vi "Steering Math.vi"() -> ()   [LabVIEW 2020]
uses:
  <vilib>/Analysis/coordinate.llb/Angle Range (Degree).ctl
  <vilib>/Analysis/coordinate.llb/Angle Units.ctl
  <vilib>/Analysis/coordinate.llb/Bisect Angle (array).vi
  <vilib>/Analysis/coordinate.llb/Angle Rotation (array).vi
  <vilib>/Analysis/coordinate.llb/Absolute Angle Difference (array).vi
  <vilib>/Analysis/coordinate.llb/Angle Rotation (scalar).vi
  <vilib>/Analysis/coordinate.llb/Wrap Angle (array).vi
  <vilib>/Analysis/coordinate.llb/Set Angle Unit.vi
  <vilib>/Analysis/coordinate.llb/Wrap Angle (scalar).vi
  <vilib>/Analysis/NI_AAL_Angle.lvlib
  <vilib>/Rock Robotics/WPI/ThirdParty/REV Robotics/REVLib/Typedef/Spark MAX Control Type.ctl
  <vilib>/Rock Robotics/WPI/ThirdParty/REV Robotics/REVLib/Typedef/Spark MAX Sensor Type.ctl
  <vilib>/Rock Robotics/WPI/ThirdParty/Phoenix-LabVIEW/Pigeon IMU/CTRE_PigeonIMU_GetYPR.vi
panel:
  out "BL Drive":dbl
  out "BR Drive":dbl
  out "FR Drive":dbl
  in  "milliseconds to wait":u32=20
  out "FL Drive":dbl
  in  "Right X":dbl
  out "Turn Left":dbl[](array[numeric])
  out "Turn Right":dbl[](array[numeric])
  out "Drive dband":dbl
  out "Steer dband":dbl
  in  "PID 550":T1={"P Gain"=0.003, "I Gain"=0.0, "D Gain"=0.006, "F Gain"=0.0, "I Zone"=0.009999999999999997, "Min Output"=-1.0, "Max Output"=1.0} {"Max Output" min=-1.0 max=1.0 step=0.01; "Min Output" min=-1.0 max=1.0 step=0.01; "I Zone" step=0.01; "F Gain" step=0.01; "D Gain" step=0.01; "I Gain" step=0.01; "P Gain" min=0.0 step=0.01}
  out "PID FL":T2(graph)
  out "FL Steer":dbl
  out "PID FR":T2(graph)
  out "FR Steer":dbl
  out "PID BL":T2(graph)
  out "BL Steer":dbl
  out "PID BR":T2(graph)
  out "BR Steer":dbl
  in  "Gyro":bool
  in  "Manual Gyro":dbl
  in  "Left X":dbl
  in  "Left Y":dbl
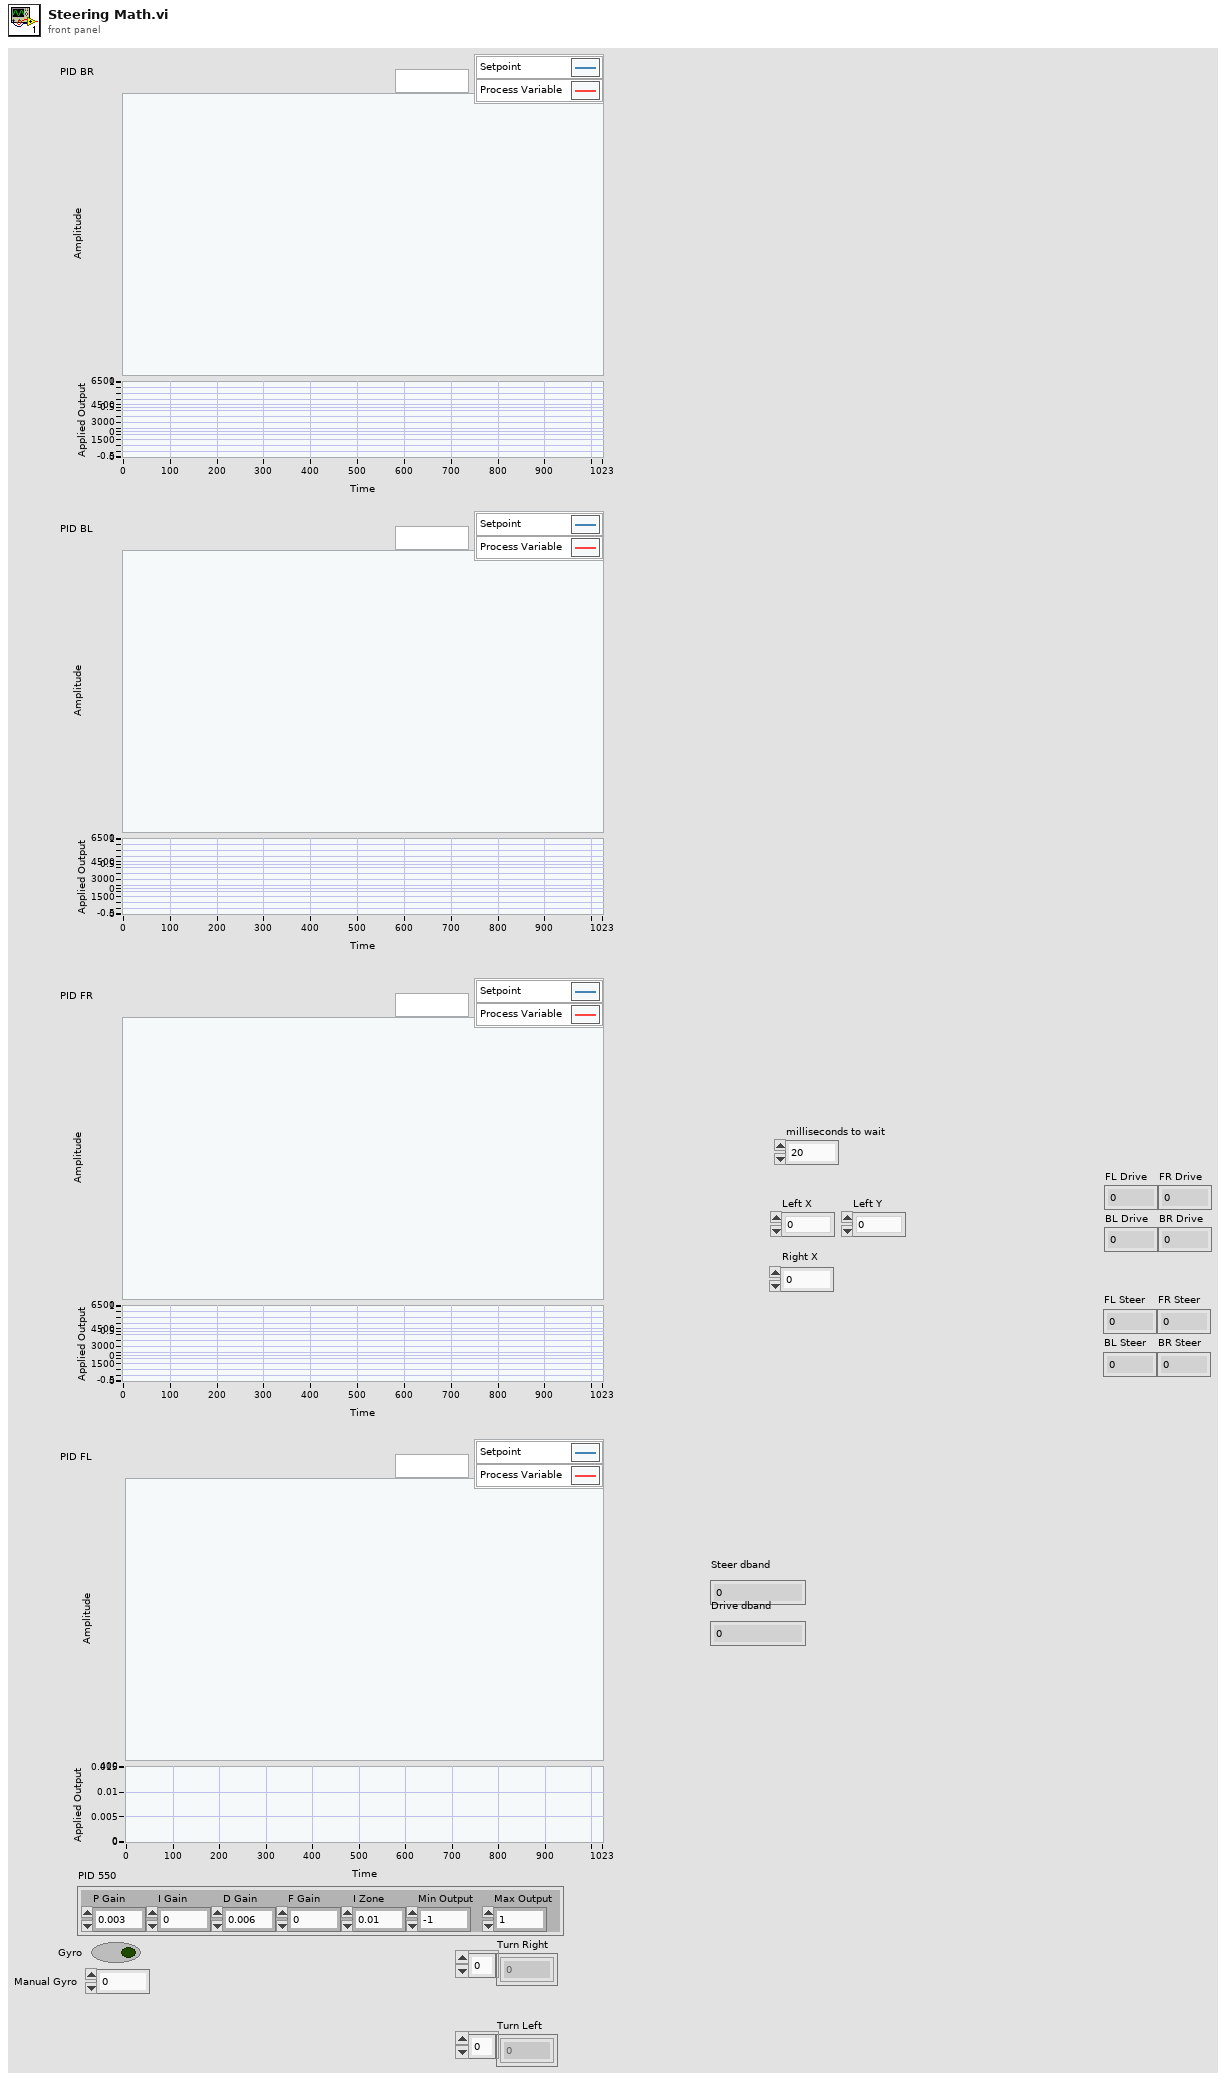
[diagram p1: front panel]
types:
  T1 = cluster{"P Gain":dbl, "I Gain":dbl, "D Gain":dbl, "F Gain":dbl, "I Zone":dbl, "Min Output":dbl, "Max Output":dbl}
  T2 = cluster{"Sensor Velocity":dbl, "Setpoint":dbl, "Applied Output":dbl}
  T3 = typedef "Spark MAX Sensor Type.ctl" = enum16{"No Sensor", "Hall Sensor", "Encoder", "-Not Available-", "Analog", "Alternate Encoder", "Duty Cycle"}
  T4 = typedef "Spark MAX Control Type.ctl" = enum16{"Percent VBus", "Voltage", "Velocity", "Position", "Smart Motion", "Current", "Smart Velocity"}
  T5 = typedef "WPI_MotorControlDeviceRef.ctl" = cluster{"DeviceStatus":errorcluster, "Type":T6, "PWM":cluster{"PWM Channel":T7, "DeadBand":T8}, "CAN":cluster{"Device Number":u8, "SetOutput VI Ref":variant, "GetOutput VI Ref":variant, "Enable VI Ref":variant, "Disable VI Ref":variant, "Data":variant}, "Invert":bool, "DIO PWM":cluster{"PWM \"Enable\" Channel":T7, "DIOChannel":T9, "PWM Rate":dbl}}
  T6 = typedef "WPI_MotorControlType.ctl" = enum16{"PWM", "CAN", "DIO PWM"}
  T7 = typedef "FPGA_DIOPWMChannel.ctl" = enum8{"PWM 0", "PWM 1", "PWM 2", "PWM 3", "PWM 4", "PWM 5", "PWM 6", "PWM 7", "PWM 8", "PWM 9", "PWM MXP 0", "PWM MXP 1", "PWM MXP 2", "PWM MXP 3", "PWM MXP 4", "PWM MXP 5", "PWM MXP 6", "PWM MXP 7", "PWM MXP 8", "PWM MXP 9", "Invalid"}
  T8 = typedef "WPI_PWMDeadband.ctl" = cluster{"Name":string, "maxPositivePwm":i32, "minPositivePwm":i32, "centerPwm":i32, "maxNegativePwm":i32, "minNegativePwm":i32, "angularRange":u16}
  T9 = typedef "FPGA_DIOChannel.ctl" = enum8{"DIO 0", "DIO 1", "DIO 2", "DIO 3", "DIO 4", "DIO 5", "DIO 6", "DIO 7", "DIO 8", "DIO 9", "DIO MXP 0", "DIO MXP 1", "DIO MXP 2", "DIO MXP 3", "DIO MXP 4", "DIO MXP 5", "DIO MXP 6", "DIO MXP 7", "DIO MXP 8", "DIO MXP 9", "DIO MXP 10", "DIO MXP 11", "DIO MXP 12", "DIO MXP 13", "DIO MXP 14", "DIO MXP 15", "SPI Port CS1", "SPI Port CS2", "SPI Port CS3", "SPI Port MISO", "SPI Port MOSI", "Invalid"}
  T10 = cluster{"P Gain":bool, "I Gain":bool, "D Gain":bool, "F Gain":bool, "I Zone":bool, "Min Output":bool, "Max Output":bool}
  T11 = cluster{"Position":dbl, void, "Applied Output":dbl}
  T12 = typedef "NI_AAL_Angle.lvlib/Angle Units.ctl" = i32
  T13 = typedef "NI_AAL_Angle.lvlib/Angle Range (Degree).ctl" = u16
  T14 = typedef "CTRE_PigeonIMU_DeviceRef.ctl" = cluster{"DeviceStatus":errorcluster, "Device Number":u8, "Type":T15, "Device ID":u32, "Handle":u64, "UsageFrame":u32, "Library Path":path}
  T15 = typedef "CTRE_PigeonIMU_ConnectionType.ctl" = u32
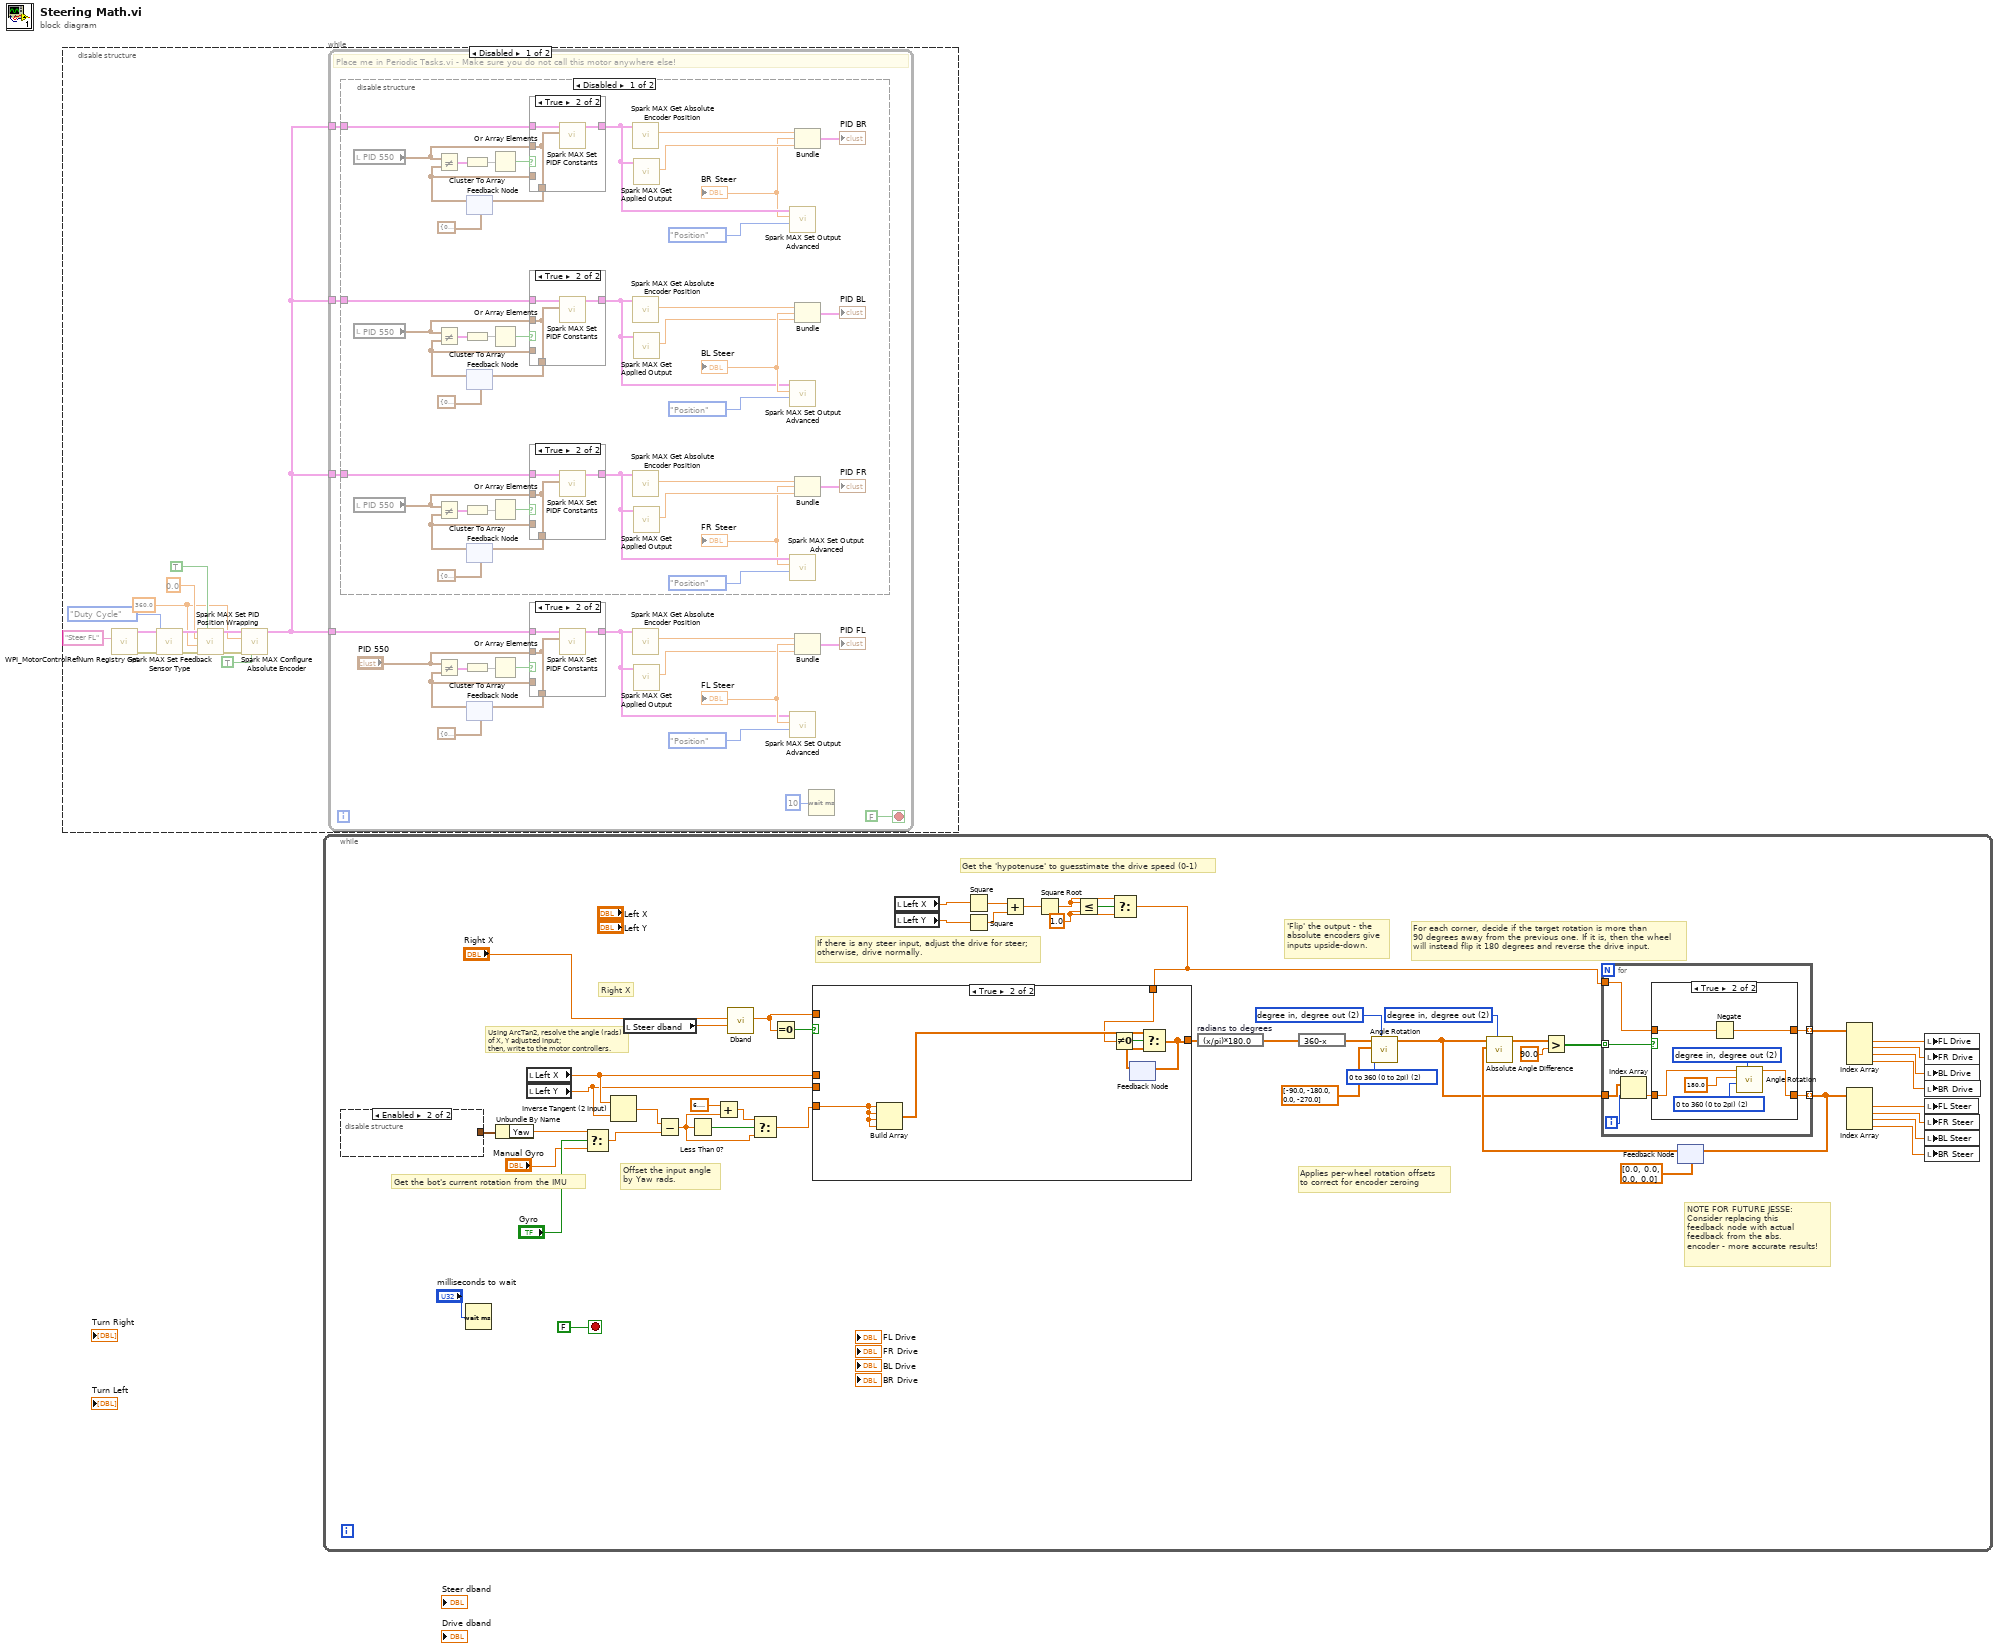
[diagram p0: block diagram]
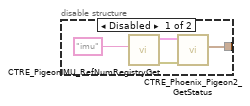
[diagram p9: hidden frame]
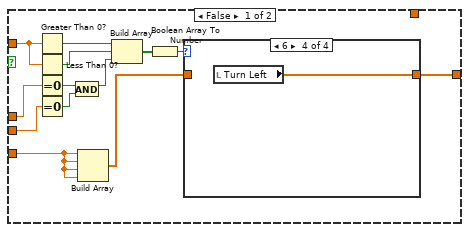
[diagram p10: hidden frame]
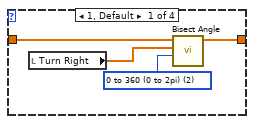
[diagram p11: hidden frame]
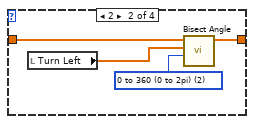
[diagram p12: hidden frame]
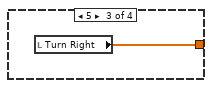
[diagram p13: hidden frame]
diagram:
  n1 = disable-structure shown="Disabled" {
    frame Disabled {
      w3 = 360.0
      n2 = call <vilib>:"WPI_MotorControlRefNum Registry Get.vi"("refnum name"="Steer FL" ("Change to match from begin.vi")) -> ("error out"=w12:errorcluster, "MotorControlDevRef"=w10:T5)  [unwired: 9 in]
      n3 = call <vilib>:"Spark MAX Set Feedback Sensor Type.vi"("error in (no error)"=w12, "Sensor Type"=Spark_MAX_Sensor_Type."Duty Cycle", "MotorControlDevRef"=w10) -> ("error out"=w11:errorcluster, "MotorControlDeviceRef"=w9:T5)  [unwired: 7 in]
      n4 = call <vilib>:"Spark MAX Set PID Position Wrapping.vi"("Enable (F)"=TRUE, "error in (no error)"=w11, "Maximum Output (0)"=w3, "Minimum Input (0)"=0.0, "MotorControlDeviceRef in"=w9) -> ("error out"=w6:errorcluster, "MotorControlDeviceRef out"=w5:T5)  [unwired: 5 in]
      n5 = call <vilib>:"Spark MAX Configure Absolute Encoder.vi"("Inverted (F)"=TRUE, "error in (no error)"=w6, "Position Conversion Factor (1)"=w3, "MotorControlDeviceRef in"=w5) -> ("MotorControlDeviceRef out"=w1:T5)  [unwired: 6 in, 1 out]
      n6 = while {
        tunnel: w1 -> [w17]
        tunnel: w1 -> [w16]
        tunnel: w1 -> [w15]
        tunnel: w1 -> [w14]
        stop <- FALSE stop-if-true
        # "Place me in Periodic Tasks.vi - Make sure you do not call this motor anywhere else!"
        n7 = disable-structure shown="Disabled" {
          disable-tunnel: w16 -> [w61 _]
          disable-tunnel: w15 -> [w60 _]
          disable-tunnel: w14 -> [w33 _]
          frame Disabled {
            n8 = local read "PID 550"() -> (w34:T1)
            n9 = local read "PID 550"() -> (w59:T1)
            n10 = local read "PID 550"() -> (w62:T1)
            n11 = feedback #1(T1 {"P Gain"=0.0, "I Gain"=0.0, "D Gain"=0.0, "F Gain"=0.0, "I Zone"=0.0, "Min Output"=0.0, "Max Output"=0.0} ("PID Constants")) -> (w38:T1)
            n12 = Not Equal?(x=w34, y=w38) -> (x != y?=w43:T10)
            n13 = Cluster To Array(cluster=w43) -> (array=w42:bool[])
            n14 = feedback #2(T1 {"P Gain"=0.0, "I Gain"=0.0, "D Gain"=0.0, "F Gain"=0.0, "I Zone"=0.0, "Min Output"=0.0, "Max Output"=0.0} ("PID Constants")) -> (w55:T1)
            n15 = Not Equal?(x=w59, y=w55) -> (x != y?=w50:T10)
            n16 = Cluster To Array(cluster=w50) -> (array=w51:bool[])
            n17 = feedback #3(T1 {"P Gain"=0.0, "I Gain"=0.0, "D Gain"=0.0, "F Gain"=0.0, "I Zone"=0.0, "Min Output"=0.0, "Max Output"=0.0} ("PID Constants")) -> (w66:T1)
            n18 = Not Equal?(x=w62, y=w66) -> (x != y?=w71:T10)
            n19 = Cluster To Array(cluster=w71) -> (array=w70:bool[])
            n20 = Or Array Elements(Boolean array=w42) -> (logical OR=w40:bool)
            n21 = Or Array Elements(Boolean array=w51) -> (logical OR=w53:bool)
            n22 = Or Array Elements(Boolean array=w70) -> (logical OR=w68:bool)
            n23 = case shown="True" w40 {
              tunnel: w33 -> [w75 w79]
              tunnel: w34 -> [_ w77]
              tunnel: [w76 w77] -> w39
              tunnel: w38 -> [w76 _]
              tunnel: [w75 w78] -> w46
              frame False {
              }
              frame True {
                n24 = call <vilib>:"Spark MAX Set PIDF Constants.vi"("PID Constants"=w77, "MotorControlDeviceRef"=w79) -> ("MotorControlDeviceRef"=w78:T5)  [unwired: 8 in, 1 out]
              }
            }
            n25 = feedback-in #1(w39) -> ()
            n26 = case shown="True" w53 {
              tunnel: w60 -> [w80 w84]
              tunnel: w59 -> [_ w82]
              tunnel: [w81 w82] -> w54
              tunnel: w55 -> [w81 _]
              tunnel: [w80 w83] -> w47
              frame False {
              }
              frame True {
                n27 = call <vilib>:"Spark MAX Set PIDF Constants.vi"("PID Constants"=w82, "MotorControlDeviceRef"=w84) -> ("MotorControlDeviceRef"=w83:T5)  [unwired: 8 in, 1 out]
              }
            }
            n28 = feedback-in #2(w54) -> ()
            n29 = case shown="True" w68 {
              tunnel: w61 -> [w85 w89]
              tunnel: w62 -> [_ w87]
              tunnel: [w86 w87] -> w67
              tunnel: w66 -> [w86 _]
              tunnel: [w85 w88] -> w74
              frame False {
              }
              frame True {
                n30 = call <vilib>:"Spark MAX Set PIDF Constants.vi"("PID Constants"=w87, "MotorControlDeviceRef"=w89) -> ("MotorControlDeviceRef"=w88:T5)  [unwired: 8 in, 1 out]
              }
            }
            n31 = feedback-in #3(w67) -> ()
            n32 = call <vilib>:"Spark MAX Get Absolute Encoder Position.vi"("MotorControlDeviceRef in"=w46) -> ("Position"=w44:dbl)  [unwired: 7 in, 3 out]
            n33 = call <vilib>:"Spark MAX Get Absolute Encoder Position.vi"("MotorControlDeviceRef in"=w47) -> ("Position"=w49:dbl)  [unwired: 7 in, 3 out]
            n34 = call <vilib>:"Spark MAX Get Absolute Encoder Position.vi"("MotorControlDeviceRef in"=w74) -> ("Position"=w72:dbl)  [unwired: 7 in, 3 out]
            n35 = call <vilib>:"Spark MAX Get Applied Output.vi"("MotorControlDevRef in"=w46) -> ("Applied Output"=w45:dbl)  [unwired: 7 in, 3 out]
            n36 = call <vilib>:"Spark MAX Get Applied Output.vi"("MotorControlDevRef in"=w47) -> ("Applied Output"=w48:dbl)  [unwired: 7 in, 3 out]
            n37 = call <vilib>:"Spark MAX Get Applied Output.vi"("MotorControlDevRef in"=w74) -> ("Applied Output"=w73:dbl)  [unwired: 7 in, 3 out]
            n38 = call <vilib>:"Spark MAX Set Output Advanced.vi"("Control Mode"=Spark_MAX_Control_Type."Position", "Setpoint"="BR Steer", "MotorControlDevRef"=w46) -> ()  [unwired: 7 in, 2 out]
            n39 = call <vilib>:"Spark MAX Set Output Advanced.vi"("Control Mode"=Spark_MAX_Control_Type."Position", "Setpoint"="BL Steer", "MotorControlDevRef"=w47) -> ()  [unwired: 7 in, 2 out]
            n40 = call <vilib>:"Spark MAX Set Output Advanced.vi"("Control Mode"=Spark_MAX_Control_Type."Position", "Setpoint"="FR Steer", "MotorControlDevRef"=w74) -> ()  [unwired: 7 in, 2 out]
            n41 = Bundle("Position"=w44, "BR Steer", "Applied Output"=w45) -> (→"PID BR":T11)  [unwired: 1 in]
            n42 = Bundle("Position"=w49, "BL Steer", "Applied Output"=w48) -> (→"PID BL":T11)  [unwired: 1 in]
            n43 = Bundle("Position"=w72, "FR Steer", "Applied Output"=w73) -> (→"PID FR":T11)  [unwired: 1 in]
          }
          frame Enabled {
          }
        }
        n44 = feedback #4(T1 {"P Gain"=0.0, "I Gain"=0.0, "D Gain"=0.0, "F Gain"=0.0, "I Zone"=0.0, "Min Output"=0.0, "Max Output"=0.0} ("PID Constants")) -> (w29:T1)
        n45 = Not Equal?(x="PID 550", y=w29) -> (x != y?=w23:T10)
        n46 = Cluster To Array(cluster=w23) -> (array=w24:bool[])
        n47 = Or Array Elements(Boolean array=w24) -> (logical OR=w26:bool)
        n48 = case shown="True" w26 {
          tunnel: w17 -> [w90 w94]
          tunnel: "PID 550" -> [_ w92]
          tunnel: [w91 w92] -> w28
          tunnel: w29 -> [w91 _]
          tunnel: [w90 w93] -> w18
          frame False {
          }
          frame True {
            n49 = call <vilib>:"Spark MAX Set PIDF Constants.vi"("PID Constants"=w92, "MotorControlDeviceRef"=w94) -> ("MotorControlDeviceRef"=w93:T5)  [unwired: 8 in, 1 out]
          }
        }
        n50 = feedback-in #4(w28) -> ()
        n51 = call <vilib>:"Spark MAX Get Absolute Encoder Position.vi"("MotorControlDeviceRef in"=w18) -> ("Position"=w20:dbl)  [unwired: 7 in, 3 out]
        n52 = call <vilib>:"Spark MAX Get Applied Output.vi"("MotorControlDevRef in"=w18) -> ("Applied Output"=w19:dbl)  [unwired: 7 in, 3 out]
        n53 = call <vilib>:"Spark MAX Set Output Advanced.vi"("Control Mode"=Spark_MAX_Control_Type."Position", "Setpoint"="FL Steer", "MotorControlDevRef"=w18) -> ()  [unwired: 7 in, 2 out]
        n54 = Bundle("Position"=w20, "FL Steer", "Applied Output"=w19) -> (→"PID FL":T11)  [unwired: 1 in]
        n55 = Wait (ms)(milliseconds to wait=u32 10) -> ()  [unwired: 1 out]
      }
    }
    frame Enabled {
    }
  }
  n56 = while {
    stop <- FALSE stop-if-true
    w105 = T12 2 items=["radian in, radian out", "radian in, degree out", "degree in, degree out", "degree in, radian out"] ("angle units")
    w102 = T12 2 items=["radian in, radian out", "radian in, degree out", "degree in, degree out", "degree in, radian out"] ("angle units")
    w103 = T13 2 items=["none", "-180 to 180 (-pi to pi)", "0 to 360 (0 to 2pi)"] ("rotated angle range")
    w137 = 1.0 ("x")
    # "NOTE FOR FUTURE JESSE:\nConsider replacing this\nfeedback node with actual\nfeedback from the abs.\nencoder - more accurate results!"
    # "'Flip' the output - the\nabsolute encoders give\ninputs upside-down."
    # "Applies per-wheel rotation offsets\nto correct for encoder zeroing"
    # "For each corner, decide if the target rotation is more than\n90 degrees away from the previous one. If it is, then the wheel\nwill instead flip it 180 degrees and reverse the drive input."
    # "Right X"
    # "If there is any steer input, adjust the drive for steer;\notherwise, drive normally."
    # "Using ArcTan2, resolve the angle (rads) of X, Y adjusted input; \nthen, write to the motor controllers."
    # "Offset the input angle\nby Yaw rads."
    # "Get the bot's current rotation from the IMU"
    # "Get the 'hypotenuse' to guesstimate the drive speed (0-1)"
    n57 = disable-structure shown="Enabled" {
      disable-tunnel: [w162 _] -> w143
      frame Disabled {
        n58 = call <vilib>:"CTRE_PigeonIMU_RefNumRegistryGet.vi"("refnum name"="imu") -> ("error out"=w164:errorcluster, "PigeonIMUDevRef"=w163:T14)  [unwired: 9 in]
        n59 = call-poly <vilib>:"CTRE_Phoenix_Pigeon2_GetStatus.vi"("error in (no error)"=w164, "PigeonIMUDevRef"=w163) -> ("Yaw Pitch Roll"=w162:cluster{"Yaw":dbl, "Pitch":dbl, "Roll":dbl})  [unwired: 7 in, 2 out]
      }
      frame Enabled {
      }
    }
    n60 = Wait (ms)(milliseconds to wait="milliseconds to wait") -> ()  [unwired: 1 out]
    n61 = Unbundle By Name(w143) -> ("Yaw"=w129:dbl)
    n62 = local read "Left X"() -> (w123:dbl)
    n63 = local read "Left Y"() -> (w122:dbl)
    n64 = Select(t=w129, s="Gyro", f="Manual Gyro") -> (s? t:f=w128:dbl)
    n65 = Inverse Tangent (2 Input)(1:w122, 2:w123) -> (0:w132:dbl)
    n66 = local read "Steer dband"() -> (w126:dbl)
    n67 = Subtract(x=w132, y=w128) -> (x-y=w136:dbl)
    n68 = Less Than 0?(x=w136) -> (x < 0?=w133:bool)
    n69 = Add(x=6.283185307179586, y=w136) -> (x+y=w134:dbl)
    n70 = call "Dband.vi"("dband"=w126, "Numeric"="Right X") -> ("Fixed"=w124:dbl)  [unwired: 9 in]
    n71 = Select(t=w134, s=w133, f=w136) -> (s? t:f=w131:dbl)
    n72 = Equal To 0?(x=w124) -> (x = 0?=w125:bool)
    n73 = local read "Left X"() -> (w121:dbl)
    n74 = local read "Left Y"() -> (w120:dbl)
    n75 = Square(x=w121) -> (x^2=w141:dbl)
    n76 = Square(x=w120) -> (x^2=w140:dbl)
    n77 = Add(x=w141, y=w140) -> (x+y=w142:dbl)
    n78 = Square Root(x=w142) -> (sqrt(x)=w138:dbl)
    n79 = Less Or Equal?(x=w138, y=w137) -> (x <= y?=w139:bool)
    n80 = Select(t=w138, s=w139, f=w137) -> (s? t:f=w97:dbl)
    n81 = case shown="True" w125 {
      tunnel: w124 -> [w178 _]
      tunnel: w123 -> [w172 _]
      tunnel: w122 -> [w171 _]
      tunnel: w131 -> [w168 w191]
      tunnel: [w166 w190] -> w98
      tunnel: w97 -> [_ w192]
      frame False {
        n82 = Greater Than 0?(x=w178) -> (x > 0?=w176:bool)
        n83 = Less Than 0?(x=w178) -> (x < 0?=w175:bool)
        n84 = Equal To 0?(x=w172) -> (x = 0?=w174:bool)
        n85 = Equal To 0?(x=w171) -> (x = 0?=w169:bool)
        n86 = And(x=w174, y=w169) -> (x .and. y?=w170:bool)
        n87 = Build Array(w168, w168, w168, w168) -> (w167:dbl[])
        n88 = Build Array(w176, w175, w170) -> (w173:bool[])
        n89 = Boolean Array To Number(Boolean array=w173) -> (number=w177:u32)
        n90 = case shown="6" w177 {
          tunnel: w167 -> [w180 w184 _ _]
          tunnel: [w179 w183 w187 w188] -> w166
          frame 1, Default {
            w182 = T13 2 items=["none", "-180 to 180 (-pi to pi)", "0 to 360 (0 to 2pi)"] ("angle bisector range")
            n91 = local read "Turn Right"() -> (w181:dbl[])
            n92 = call-poly <vilib>:"Bisect Angle.vi"("angle bisector range"=w182, "End Angle"=w181, "Start Angle"=w180) -> ("Angle Bisector"=w179:dbl[])  [unwired: 7 in, 1 out]
          }
          frame 2 {
            w186 = T13 2 items=["none", "-180 to 180 (-pi to pi)", "0 to 360 (0 to 2pi)"] ("angle bisector range")
            n93 = local read "Turn Left"() -> (w185:dbl[])
            n94 = call-poly <vilib>:"Bisect Angle.vi"("angle bisector range"=w186, "End Angle"=w185, "Start Angle"=w184) -> ("Angle Bisector"=w183:dbl[])  [unwired: 7 in, 1 out]
          }
          frame 5 {
            n95 = local read "Turn Right"() -> (w187:dbl[])
          }
          frame 6 {
            n96 = local read "Turn Left"() -> (w188:dbl[])
          }
        }
      }
      frame True {
        n97 = Build Array(w191, w191, w191, w191) -> (w194:dbl[])
        n98 = Not Equal To 0?(x=w192) -> (x != 0?=w193:bool)
        n99 = feedback #5() -> (w189:dbl[])  [unwired: 1 in]
        n100 = Select(t=w194, s=w193, f=w189) -> (s? t:f=w190:dbl[])
        n101 = feedback-in #5(w190) -> ()
      }
    }
    n102 = expression code="(x/pi)*180.0" "radians to degrees"(w98) -> (w95:dbl[])
    n103 = expression code="360-x"(w95) -> (w104:dbl[])
    n104 = call-poly <vilib>:"Angle Rotation.vi"("angle units"=w102, "rotated angle range"=w103, "Counterclockwise Rotation"=dbl[] [-90.0, -180.0, 0.0, -270.0], "Angle"=w104) -> ("Rotated Angle"=w109:dbl[])  [unwired: 6 in, 1 out]
    n105 = feedback #6(dbl[] [0.0, 0.0, 0.0, 0.0]) -> (w110:dbl[])
    n106 = call-poly <vilib>:"Absolute Angle Difference.vi"("angle units"=w105, "Angle 2"=w110, "Angle 1"=w109) -> ("Absolute Angle Difference"=w106:dbl[])  [unwired: 7 in, 1 out]
    n107 = Greater?(x=w106, y=90.0) -> (0:w108:bool[])
    n108 = for {
      tunnel: w108 -> [w152] mode=indexing
      tunnel: w109 -> [w149]
      tunnel: [w148] -> w99 mode=indexing
      tunnel: [w150] -> w100 mode=indexing
      tunnel: w97 -> [w147]
      i -> [w146]
      n109 = Index Array(array=w149, index=w146) -> (element=w151:dbl)
      n110 = case shown="True" w152 {
        tunnel: w151 -> [w154 w159]
        tunnel: [w154 w157] -> w150
        tunnel: w147 -> [w153 w156]
        tunnel: [w153 w155] -> w148
        frame False {
        }
        frame True {
          w160 = T13 2 items=["none", "-180 to 180 (-pi to pi)", "0 to 360 (0 to 2pi)"] ("rotated angle range")
          w161 = T12 2 items=["radian in, radian out", "radian in, degree out", "degree in, degree out", "degree in, radian out"] ("angle units")
          n111 = Negate(x=w156) -> (-x=w155:dbl)
          n112 = call-poly <vilib>:"Angle Rotation.vi"("angle units"=w161, "rotated angle range"=w160, "counterclockwise rotation"=180.0, "angle"=w159) -> ("rotated angle"=w157:dbl)  [unwired: 6 in, 1 out]
        }
      }
    }
    n113 = feedback-in #6(w100) -> ()
    n114 = Index Array(array=w99) -> (element #1=w111:dbl, element #2=w112:dbl, element #3=w113:dbl, element #4=w114:dbl)  [unwired: 4 in]
    n115 = Index Array(array=w100) -> (element #1=w118:dbl, element #2=w117:dbl, element #3=w116:dbl, element #4=w115:dbl)  [unwired: 4 in]
    n116 = local write "FL Drive"(w111) -> ()
    n117 = local write "FR Drive"(w112) -> ()
    n118 = local write "BL Drive"(w113) -> ()
    n119 = local write "BR Drive"(w114) -> ()
    n120 = local write "FL Steer"(w118) -> ()
    n121 = local write "FR Steer"(w117) -> ()
    n122 = local write "BL Steer"(w116) -> ()
    n123 = local write "BR Steer"(w115) -> ()
  }
